vi "Identify Blob.vi"(10 "Particle Report":T1) -> (2 "Result":string)   [LabVIEW 2013]
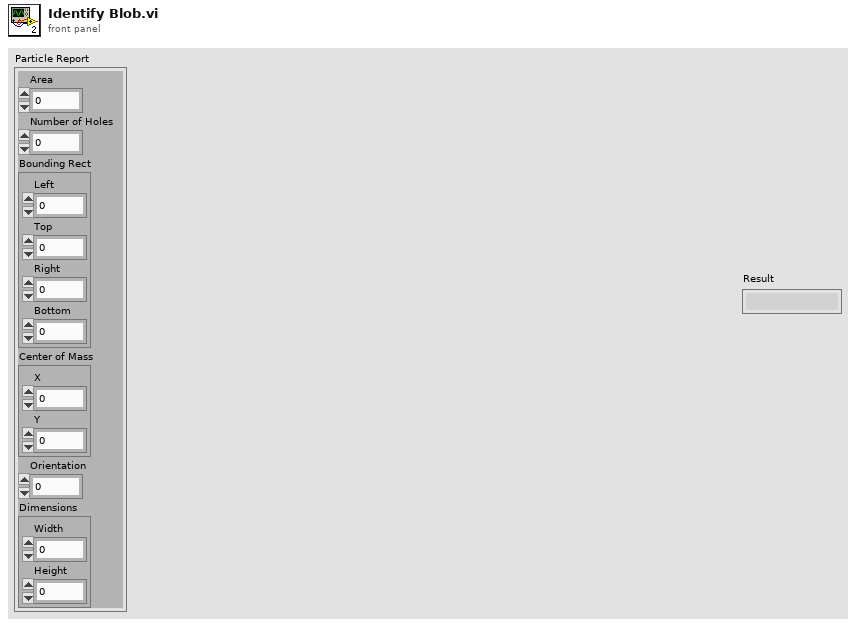
[diagram p1: front panel]
types:
  T1 = cluster{"Area":dbl, "Number of Holes":dbl, "Bounding Rect":cluster{"Left":dbl, "Top":dbl, "Right":dbl, "Bottom":dbl}, "Center of Mass":cluster{"X":dbl, "Y":dbl}, "Orientation":dbl, "Dimensions":cluster{"Width":dbl, "Height":dbl}}
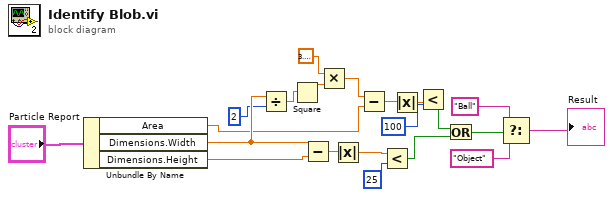
[diagram p0: block diagram]
diagram:
  n1 = Unbundle By Name("Particle Report") -> ("Area"=w10:dbl, "Dimensions.Width"=w16:dbl, "Dimensions.Height"=w17:dbl)
  n2 = Divide(x=w16, y=2) -> (x/y=w14:dbl)
  n3 = Square(x=w14) -> (x^2=w13:dbl)
  n4 = Subtract(x=w16, y=w17) -> (x-y=w20:dbl)
  n5 = Multiply(x=3.141592653589793, y=w13) -> (x*y=w11:dbl)
  n6 = Absolute Value(x=w20) -> (abs(x)=w19:dbl)
  n7 = Subtract(x=w11, y=w10) -> (x-y=w9:dbl)
  n8 = Less?(x=w19, y=25) -> (x < y?=w5:bool)
  n9 = Absolute Value(x=w9) -> (abs(x)=w8:dbl)
  n10 = Less?(x=w8, y=100) -> (x < y?=w6:bool)
  n11 = Or(x=w6, y=w5) -> (x .or. y?=w4:bool)
  n12 = Select(t="Ball", s=w4, f="Object") -> (s? t:f=→"Result":string)
